vi "init.vi"(8 "error in (no error)":errorcluster, 11 "PreconditioningMonitor in":refnum<class "PreconditioningMonitor.lvclass">) -> (0 "error out":errorcluster, 3 "PreconditioningMonitor out":refnum<class "PreconditioningMonitor.lvclass">)   [LabVIEW 2015, in "PreconditioningMonitor.lvclass"]
uses:
  PreconditioningMonitor.lvclass
  StiffnessCalculator/Preconditioning.ctl
  PreconditioningMonitor.lvclass/PreconditioningMonitor.ctl
  ConfigurationThisComponent/ConfigurationThisComponent.lvclass
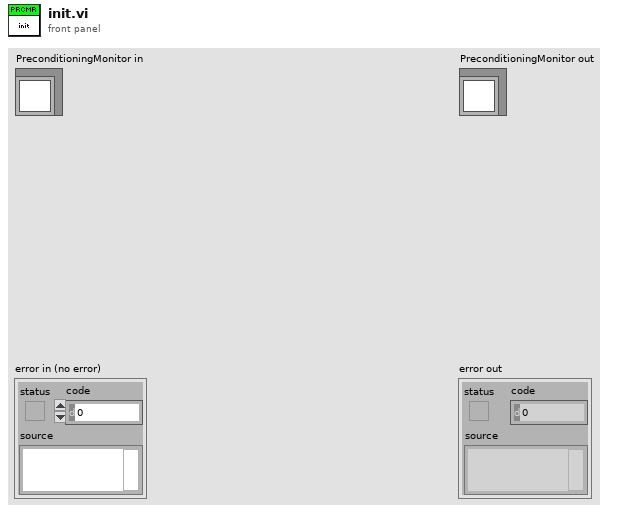
[diagram p1: front panel]
types:
  T1 = typedef "Preconditioning.ctl" = cluster{"Number of preconditioning cycles":u32}
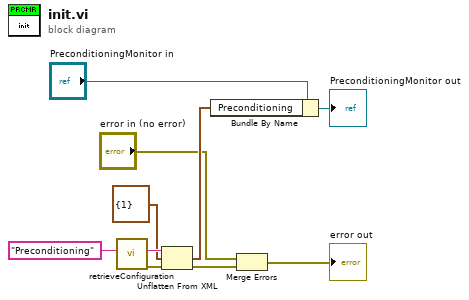
[diagram p0: block diagram]
diagram:
  n1 = call "retrieveConfiguration.vi"("configName"="Preconditioning") -> ("error out"=w8:errorcluster, "xmlConfig"=w7:string)  [unwired: 8 in, 1 out]
  n2 = Unflatten From XML(xml string=w7, type=T1 {"Number of preconditioning cycles"=1} ("Preconditioning"), error in (no error)=w8) -> (value=w5:T1, error out=w10:errorcluster)
  n3 = Bundle By Name(cluster="PreconditioningMonitor in", "Preconditioning"=w5) -> (→"PreconditioningMonitor out":refnum<class "PreconditioningMonitor.lvclass">)
  n4 = Merge Errors("error in (no error)", w10) -> (→"error out":errorcluster)
